vi "Data Access.vi"(8 "error in (no error)":errorcluster, 10 "Data Access Handler":refnum<class "Data Access Handler.lvclass">, 11 "Flex Msg in":refnum<class "Flex Msg.lvclass">) -> (0 "error out":errorcluster, 3 "Flex Msg out":refnum<class "Flex Msg.lvclass">)   [LabVIEW 2020, in "Msg.lvlib" / "Flex Msg.lvclass"]
doc: "Expose class private data to the front panel while letting the Data Access Handler class act on the data."
uses:
  Flex Msg.lvclass
  Data Access Handlers/Data Access Handler/Data Access Handler.lvclass
panel:
  in  "Cancel":bool
  in  "OK":bool
  # "No Data Access method implemented \nfor this message."
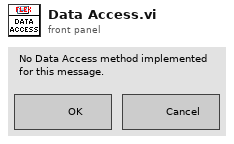
[diagram p1: front panel]
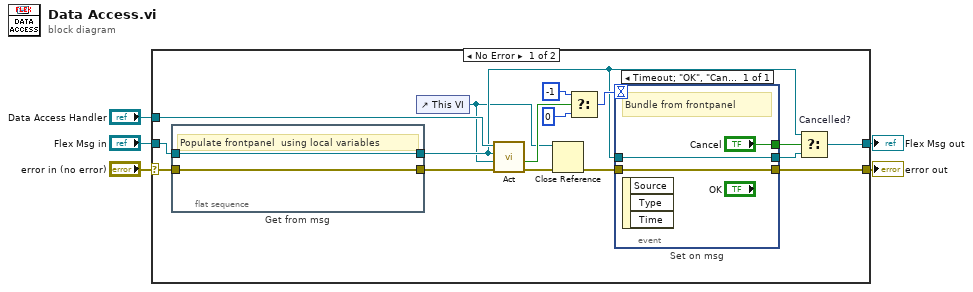
[diagram p0: block diagram]
diagram:
  n1 = case shown="No Error" "error in (no error)" {
    selector: "error in (no error)" -> [w21 w28]
    tunnel: [w14 w28] -> w4
    tunnel: [w9 w27] -> w2
    tunnel: "Flex Msg in" -> [w12 w27]
    tunnel: "Data Access Handler" -> [w20 _]
    frame No Error {
      n2 = flat-sequence "Get from msg" {
        tunnel: w21 -> [w25]
        tunnel: [w26] -> w7
        tunnel: w12 -> [w26]
        tunnel: [w25] -> w19
        frame #0 {
          # "Populate frontpanel  using local variables"
        }
      }
      n3 = control-ref of="This VI"() -> (w6:refnum<vi>)
      n4 = call-dynamic "Act.vi"("error in (no error)"=w19, "VI Refnum in"=w6, "Flex Msg type"=w7, "Data Access Handler in"=w20) -> ("error out"=w11:errorcluster, "Await user action?"=w18:bool)  [unwired: 5 in, 1 out]
      n5 = Close Reference(reference=w6, error in (no error)=w11) -> (error out=w13:errorcluster)
      n6 = Select(t=-1, s=w18, f=0 ("t")) -> (s? t:f=w15:i32)
      n7 = event "Set on msg" shown="[0] Timeout;  \"OK\", \"Cancel\": Value Change" {
        selector: _ -> [_]
        dyn-events: _ -> [_]
        timeout: w15 -> [_]
        tunnel: [w24] -> w14
        tunnel: w13 -> [w24]
        tunnel: ["Cancel"] -> w10
        tunnel: [w23] -> w8
        tunnel: w7 -> [w23]
        event Timeout; "OK", "Cancel": Value Change {
          # "Bundle from frontpanel"
          n8 = event-data() -> ()  [unwired: 1 in, 3 out]
        }
      }
      n9 = Select "Cancelled?"(t=w7, s=w10, f=w8) -> (s? t:f=w9:refnum<class "Flex Msg.lvclass">)
    }
    frame Error {
    }
  }
  "error out" <- w4
  "Flex Msg out" <- w2
